vi "convert scan cluster to file scan with multibin drift check.vi"(0 "Scan parameters":T1 {"Scan Start" format="%#.9p"; "Scan End" format="%#.9p"; "Scan Step Size" format="%#.9p"}, 1 "check value":dbl, 2 "precision (12)":i16=12, 3 "multibin":i16) -> (7 "spreadsheet string":string, 8 "values":string[](array[string]), 9 "values:numshots":string[](array[string]))   [LabVIEW 2013]
uses:
  scan parameters.ctl
  <vilib>/Analysis/1siggen.llb/Ramp Pattern by Delta.vi
  <vilib>/Analysis/NI_AALBase.lvlib
panel:
  out "Ramp Pattern":dbl[](array[numeric])
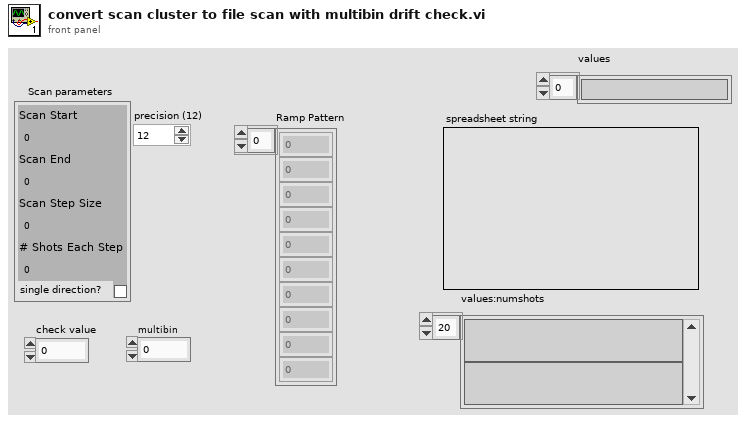
[diagram p1: front panel]
types:
  T1 = typedef "scan parameters.ctl" = cluster{"Scan Start":dbl, "Scan End":dbl, "Scan Step Size":dbl, "# Shots Each Step":u32, "single direction?":bool}
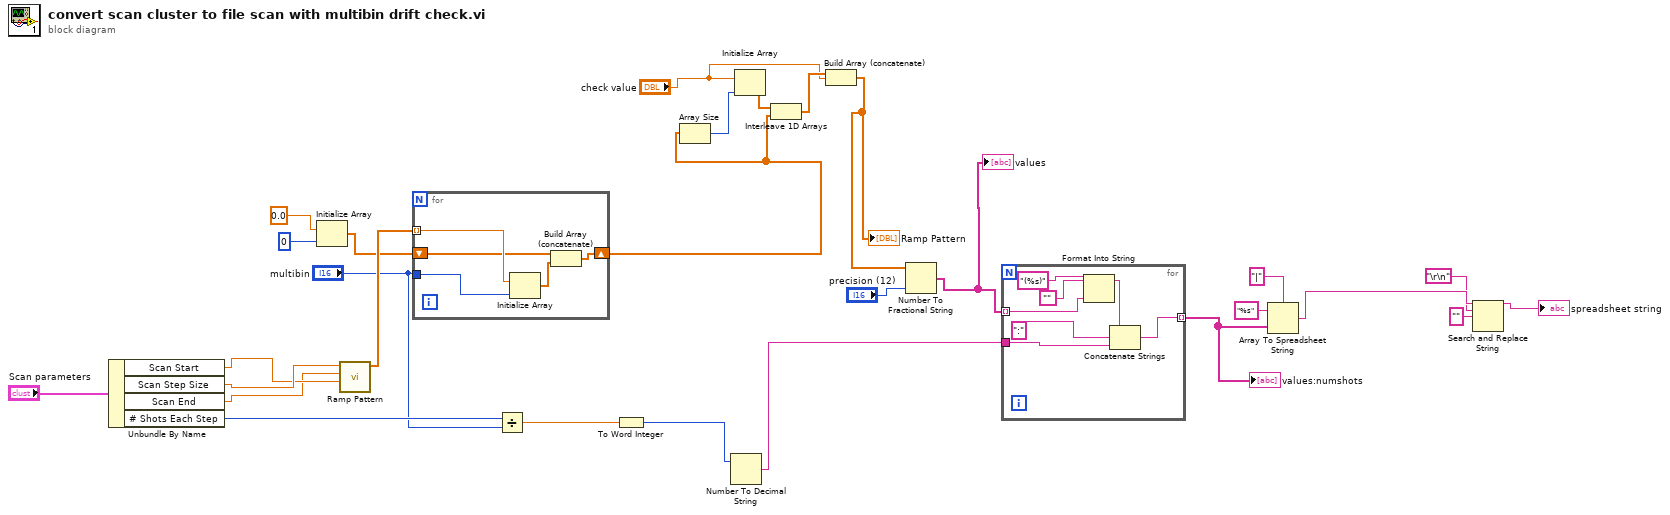
[diagram p0: block diagram]
diagram:
  n1 = Unbundle By Name("Scan parameters") -> ("Scan Start"=w26:dbl, "Scan Step Size"=w27:dbl, "Scan End"=w25:dbl, "# Shots Each Step"=w7:u32)
  n2 = Initialize Array(0.0, 0) -> (w3:dbl[])
  n3 = call-poly <vilib>:"Ramp Pattern.vi"("start"=w26, "end"=w25, "delta"=w27) -> ("Ramp Pattern"=w9:dbl[])  [unwired: 6 in, 2 out]
  n4 = for {
    tunnel: w9 -> [w32] mode=indexing
    tunnel: "multibin" -> [w33]
    shift-right: [w30] -> w8
    shift-left: w3 -> [w29]
    n5 = Initialize Array(w32, w33) -> (w31:dbl[])
    n6 = Build Array (concatenate)(w29, w31) -> (w30:dbl[])
  }
  n7 = Divide(x=w7, y="multibin") -> (x/y=w4:dbl)
  n8 = To Word Integer(number=w4) -> (16bit integer=w5:i16)
  n9 = Array Size(array=w8) -> (size(s)=w14:i32)
  n10 = Number To Decimal String(number=w5) -> (decimal integer string=w23:string)  [unwired: 1 in]
  n11 = Initialize Array("check value", w14) -> (w13:dbl[])
  n12 = Interleave 1D Arrays(w13, w8) -> (w12:dbl[])
  n13 = Build Array (concatenate)(w12, "check value") -> (w10:dbl[])
  "Ramp Pattern" <- w10
  n14 = Number To Fractional String(number=w10, precision (6)="precision (12)") -> (F-format string=w19:string[])  [unwired: 2 in]
  "values" <- w19
  n15 = for {
    tunnel: w19 -> [w35] mode=indexing
    tunnel: w23 -> [w39]
    tunnel: [w38] -> w22 mode=indexing
    n16 = Format Into String(format string="(%s)", initial string="", w35) -> (resulting string=w37:string)  [unwired: 1 in, 1 out]
    n17 = Concatenate Strings(w37, ":" ("string"), w39) -> (w38:string)
  }
  "values:numshots" <- w22
  n18 = Array To Spreadsheet String(delimiter (Tab)="|", array=w22, 3:"%s" ("format string")) -> (spreadsheet string=w18:string)
  n19 = Search and Replace String(input string=w18, search string="\r\n", replace string="" ("replace string (\"\")")) -> (result string=→"spreadsheet string":string)  [unwired: 5 in, 3 out]
